vi "判断球及反馈 (子VI).vi"(3 "找到球？":bool, 8 "下限":dbl=10000.0 format="%#_13g", 9 "步进":dbl=1000.0 format="%#_13g", 10 "初始值":dbl=30000.0 format="%#_13g") -> (11 "阈值输出":dbl)   [LabVIEW 2017, in "年前程序.lvlib"]
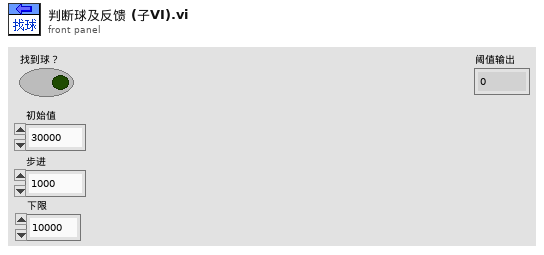
[diagram p1: front panel]
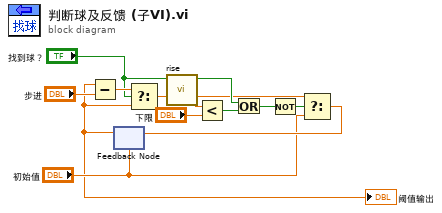
[diagram p0: block diagram]
diagram:
  n1 = feedback #1("初始值") -> (w1:dbl)
  "阈值输出" <- w1
  n2 = Subtract(x=w1, y="步进") -> (x-y=w3:dbl)
  n3 = Select(t=w3, s="找到球？", f=w1) -> (s? t:f=w6:dbl)
  n4 = call "rise.vi"("Signal"="找到球？") -> ("Count?"=w10:bool)  [unwired: 10 in]
  n5 = Less?(x=w6, y="下限") -> (x < y?=w9:bool)
  n6 = Or(x=w10, y=w9) -> (x .or. y?=w11:bool)
  n7 = Not(x=w11) -> (.not. x?=w12:bool)
  n8 = Select(t=w6, s=w12, f="初始值") -> (s? t:f=w8:dbl)
  n9 = feedback-in #1(w8) -> ()
